vi "Read Session.vi"(8 "error in (no error)":errorcluster, 11 "Camera Imaqdx in":refnum<class "Camera Imaqdx.lvclass">) -> (0 "error out":errorcluster, 2 "IMAQdx Session":T1, 3 "Camera Imaqdx out":refnum<class "Camera Imaqdx.lvclass">)   [LabVIEW 2023, in "HAL.lvlib" / "Camera Imaqdx.lvclass"]
uses:
  Camera Imaqdx.lvclass
  D:/git/HAL/Camera Base/Camera Base.lvclass
  <vilib>/userDefined/High Color/IMAQdx.ctl
  Configuration/Camera Imaqdx CFG.lvclass
  Camera Base/Camera Base.lvclass/Camera Base.ctl
  Configuration/Camera Imaqdx CFG.lvclass/Camera Imaqdx CFG.ctl
  Interfaces/IConfigure/IConfigure.lvclass
  Camera Imaqdx.lvclass/Camera Imaqdx.ctl
  Camera Base/Camera Base.lvclass
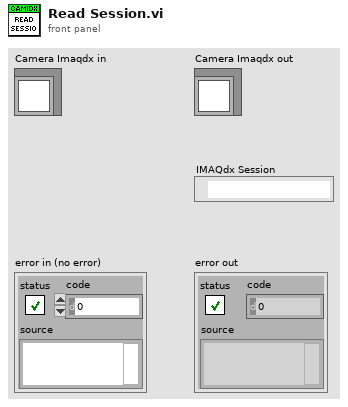
[diagram p1: front panel]
types:
  T1 = typedef "IMAQdx.ctl" = refnum<k21>
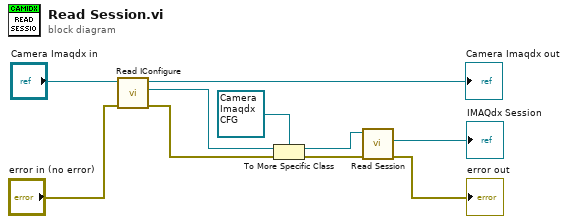
[diagram p0: block diagram]
diagram:
  n1 = call "Read IConfigure.vi"("error in (no error)"="error in (no error)", "Camera Base in"="Camera Imaqdx in") -> ("error out"=w6:errorcluster, "IConfigure"=w4:refnum<class "IConfigure.lvclass">, "Camera Base out"=→"Camera Imaqdx out":refnum<class "Camera Imaqdx.lvclass">)  [unwired: 7 in]
  n2 = To More Specific Class(target class=refnum<class "Camera Imaqdx CFG.lvclass"> refnum ("HAL.lvlib:Camera Imaqdx CFG.lvclass"), reference=w4, error in=w6) -> (specific class reference=w2:refnum<class "Camera Imaqdx CFG.lvclass">, error out=w5:errorcluster)
  n3 = call "Read Session.vi"("error in (no error)"=w5, "Camera Imaqdx CFG in"=w2) -> ("error out"=→"error out":errorcluster, "IMAQdx Session"=→"IMAQdx Session":T1)  [unwired: 7 in, 1 out]
